vi "Convert Degrees to Radians.vi"(4 "Angle (deg)":dbl) -> (1 "Angle (rad)":dbl)   [LabVIEW 2014]
doc: "Convert degrees to radians."
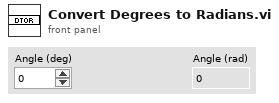
[diagram p1: front panel]
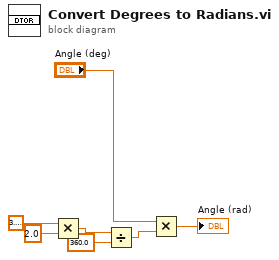
[diagram p0: block diagram]
diagram:
  n1 = Multiply(x=3.141592653589793, y=2.0) -> (x*y=w3:dbl)
  n2 = Divide(x=w3, y=360.0) -> (x/y=w5:dbl)
  n3 = Multiply(x="Angle (deg)", y=w5) -> (x*y=→"Angle (rad)":dbl)
